vi "Configure Clock Recovery.vi"(5 "Clock Recovery (T: Enable)":bool=TRUE, 6 "Recovery Channel Source (1: Channel 1)":i32(ring)=1 items=["Channel 1"=1, "Channel 2"=2, "Channel 3"=3, "Channel 4"=4], 7 "Auto Vertical Scale (T: Enable)":bool=TRUE, 8 "error in (no error)":errorcluster, 9 "Vertical Range (64 V)":dbl=64.0, 10 "Vertical Offset (0 V)":dbl, 11 "VISA resource name":refnum<visa-resource-name>) -> (0 "error out":errorcluster, 3 "VISA resource name out":refnum<visa-resource-name>)   [LabVIEW 2013, in "Agilent 90000 Series.lvlib"]
doc: "Enables or disables recovered clock and configures the vertical settings."
uses:
  Agilent 90000 Series.lvlib
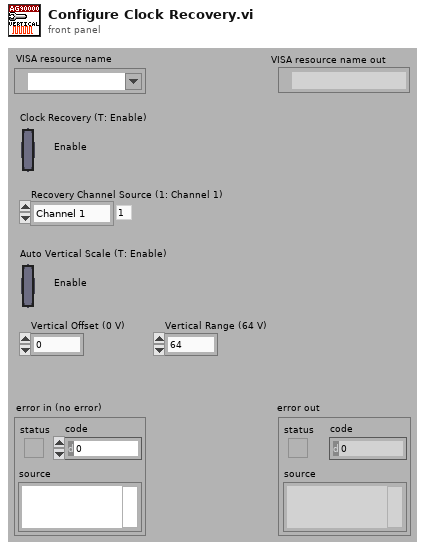
[diagram p1: front panel]
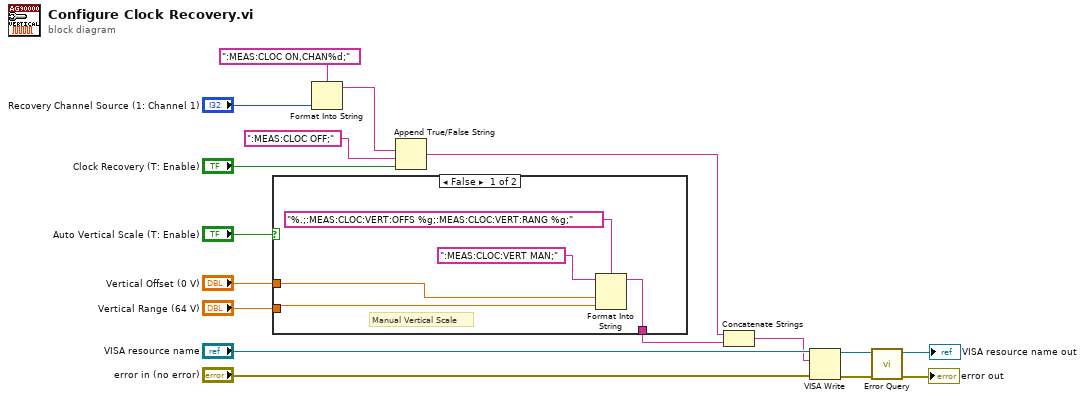
[diagram p0: block diagram]
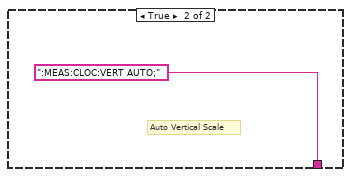
[diagram p2: hidden frame]
diagram:
  n1 = case shown="False" "Auto Vertical Scale (T: Enable)" {
    tunnel: [w18 ":MEAS:CLOC:VERT AUTO;"] -> w2
    tunnel: "Vertical Offset (0 V)" -> [w20 _]
    tunnel: "Vertical Range (64 V)" -> [w19 _]
    frame False {
      # "Manual Vertical Scale"
      n2 = Format Into String(format string="%.;:MEAS:CLOC:VERT:OFFS %g;:MEAS:CLOC:VERT:RANG %g;" ("Manual Vertical Offset and Range"), initial string=":MEAS:CLOC:VERT MAN;", w20, w19) -> (resulting string=w18:string)  [unwired: 1 in, 1 out]
    }
    frame True {
      # "Auto Vertical Scale"
    }
  }
  n3 = Format Into String(format string=":MEAS:CLOC ON,CHAN%d;", "Recovery Channel Source (1: Channel 1)") -> (resulting string=w6:string)  [unwired: 2 in, 1 out]
  n4 = Append True/False String(1:"Clock Recovery (T: Enable)", 2:":MEAS:CLOC OFF;" ("format string"), 3:w6) -> (0:w3:string)  [unwired: 1 out]
  n5 = Concatenate Strings(w3, w2) -> (w1:string)
  n6 = VISA Write(VISA resource name="VISA resource name", write buffer=w1, error in (no error)="error in (no error)") -> (VISA resource name out=w15:refnum<visa-resource-name>, error out=w14:errorcluster)  [unwired: 1 out]
  n7 = call "Error Query.vi"("error in (no error)"=w14, "VISA resource name"=w15) -> ("error out"=→"error out":errorcluster, "VISA resource name out"=→"VISA resource name out":refnum<visa-resource-name>)  [unwired: 8 out]
